vi "Rename.vi"(8 "error in (no error)":errorcluster, 9 "New Name":string, 10 "Old Name":string, 11 "FSM.Edge in":refnum<class "FSM.Edge.lvclass">) -> (0 "error out":errorcluster, 3 "FSM.Edge out":refnum<class "FSM.Edge.lvclass">)   [LabVIEW 2015, in "FSM.Edge.lvclass"]
uses:
  FSM.Edge.lvclass
  FSM.Edge.lvclass/FSM.Edge.ctl
  FSM.Label/FSM.Label.lvclass/FSM.Label.ctl
  FSM.Label/Write Text.vi
  FSM.Label/Read Text.vi
  FSM.Label/FSM.Label.lvclass
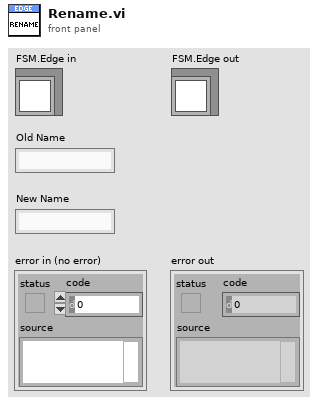
[diagram p1: front panel]
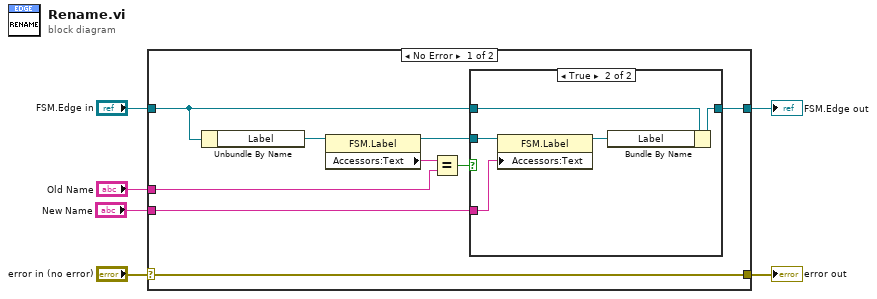
[diagram p0: block diagram]
diagram:
  n1 = case shown="No Error" "error in (no error)" {
    selector: "error in (no error)" -> [w15 w23]
    tunnel: [w15 w23] -> w5
    tunnel: [w8 w22] -> w3
    tunnel: "FSM.Edge in" -> [w10 w22]
    tunnel: "Old Name" -> [w12 _]
    tunnel: "New Name" -> [w7 _]
    frame No Error {
      n2 = Unbundle By Name(w10) -> ("Label"=w14:refnum<class "FSM.Label.lvclass">)
      n3 = property class="FSM.Label"(reference=w14) -> (reference out=w9:refnum<class "FSM.Label.lvclass">, "Accessors:Text"=w13:string)  [unwired: 1 in, 1 out]
      n4 = Equal?(x=w13, y=w12) -> (x = y?=w11:bool)
      n5 = case shown="True" w11 {
        tunnel: w10 -> [w16 w20]
        tunnel: w9 -> [_ w21]
        tunnel: [w16 w18] -> w8
        tunnel: w7 -> [_ w17]
        frame False {
        }
        frame True {
          n6 = property class="FSM.Label"(reference=w21, "Accessors:Text"=w17) -> (reference out=w19:refnum<class "FSM.Label.lvclass">)  [unwired: 1 in, 1 out]
          n7 = Bundle By Name(cluster=w20, "Label"=w19) -> (w18:refnum<class "FSM.Edge.lvclass">)
        }
      }
    }
    frame Error {
    }
  }
  "error out" <- w5
  "FSM.Edge out" <- w3
